vi "Get Transfer Group Configurations.vi"(11 "Plugin Configuration in":refnum<class "Plugin Configuration.lvclass">) -> (2 "Transfer Group Configurations":refnum<class "Transfer Group Configuration.lvclass">[](array[class]), 3 "Plugin Configuration out":refnum<class "Plugin Configuration.lvclass">)   [LabVIEW 2017, in "Data Sharing Framework Core.lvlib" / "Data Sharing Framework Engine.lvlib" / "Plugin Configuration.lvclass"]
uses:
  Plugin Configuration.lvclass
  Transfer Group Configuration/Transfer Group Configuration.lvclass
  Plugin Configuration.lvclass/Plugin Configuration.ctl
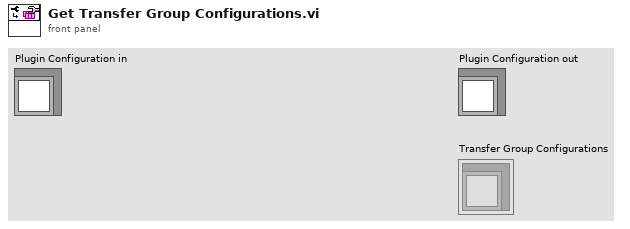
[diagram p1: front panel]
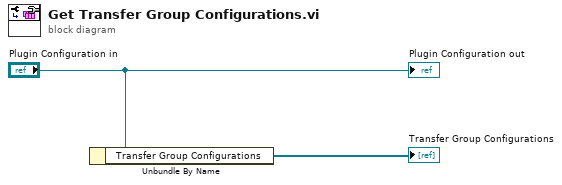
[diagram p0: block diagram]
diagram:
  n1 = Unbundle By Name("Plugin Configuration in") -> ("Transfer Group Configurations"=→"Transfer Group Configurations":refnum<class "Transfer Group Configuration.lvclass">[])
  "Plugin Configuration out" <- "Plugin Configuration in"
